vi "dvSubvi.vi"(1 "Array in":dbl[](array[numeric])) -> (0 "x-y":dbl[](array[numeric]))   [LabVIEW 2021]
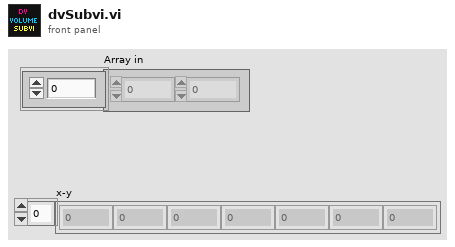
[diagram p1: front panel]
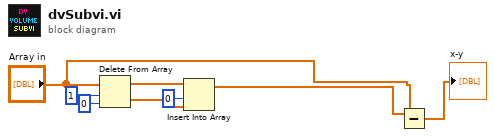
[diagram p0: block diagram]
diagram:
  n1 = Delete From Array(array="Array in", length=1, index=0) -> (deleted portion=w7:dbl[], array with subset deleted=w8:dbl[])
  n2 = Insert Into Array(array=w8, index=0, new element=w7) -> (w6:dbl[])
  n3 = Subtract(x=w6, y="Array in") -> (x-y=→"x-y":dbl[])
